vi "Read Serial.vi"() -> ()   [LabVIEW 2024]
uses:
  <vilib>/Instr/_visa.llb/VISA Configure Serial Port (Instr).vi
panel:
  out "Tank":dbl(slide) scale=0.0..1023.0
  out "Meter":dbl(knob) scale=0.0..1023.0
  out "String":string
  in  "VISA resource name":refnum<visa-resource-name>
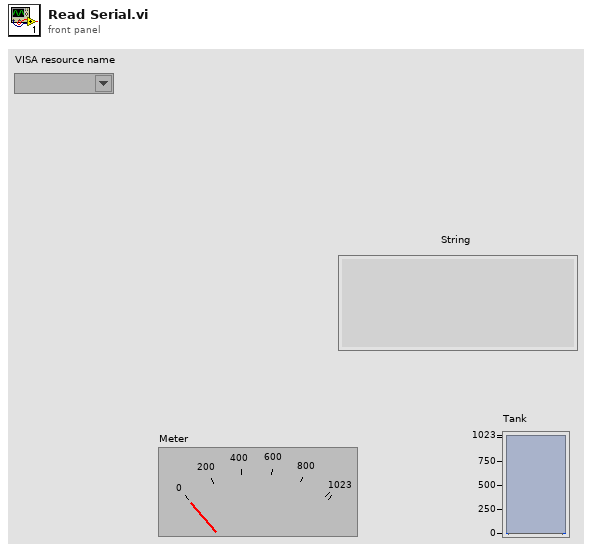
[diagram p1: front panel]
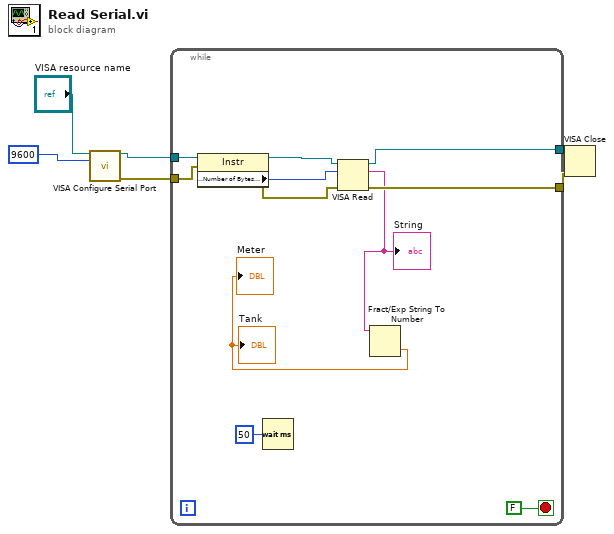
[diagram p0: block diagram]
diagram:
  n1 = call-poly "VISA Configure Serial Port"("VISA resource name"="VISA resource name", "baud rate (9600)"=u32 9600) -> ("VISA resource name out"=w6:refnum<visa-resource-name>, "error out"=w5:errorcluster)  [unwired: 12 in]
  n2 = while {
    tunnel: w6 -> [w17]
    tunnel: w5 -> [w16]
    tunnel: [w12] -> w4
    tunnel: [w11] -> w3
    stop <- FALSE stop-if-true
    n3 = property class="Instr"(reference=w17, error in=w16) -> (reference out=w14:refnum<visa-resource-name>, error out=w15:errorcluster, "Serial Settings:Number of Bytes at Serial Port"=w13:u32)
    n4 = Wait (ms)(milliseconds to wait=u32 50) -> ()  [unwired: 1 out]
    n5 = VISA Read(VISA resource name=w14, byte count=w13, error in (no error)=w15) -> (VISA resource name out=w12:refnum<visa-resource-name>, read buffer=w10:string, error out=w11:errorcluster)  [unwired: 1 out]
    "String" <- w10
    n6 = Fract/Exp String To Number(string=w10) -> (number=→"Meter" →"Tank":dbl)  [unwired: 3 in, 1 out]
  }
  n7 = VISA Close(VISA resource name=w4, error in (no error)=w3) -> ()  [unwired: 1 out]
